vi "Overlay Coordinate System.vi"(6 "Color":u32(colorbox)=16711680, 7 "Group":string, 8 "error in":errorcluster, 9 "Axis Length":i32=150, 10 "Calibration Axis Info":T2={"Origin Pixel"={"X"=0.0, "Y"=0.0}, "Angle Relative to Horizontal (deg)"=20.0, "Axis Reference"=0} {"Axis Reference" items=["Direct", "Indirect"]; "Angle Relative to Horizontal (deg)" format="%.2f"}, 11 "Image":T1) -> (0 "error out":errorcluster, 3 "Image Out":T1)   [LabVIEW 2016]
doc: "Overlay a coordinate system on the image."
uses:
  <vilib>/vision/Image Controls.llb/IMAQ Image.ctl
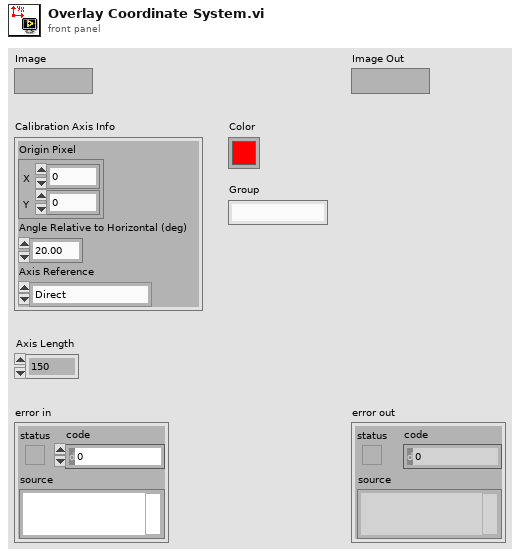
[diagram p1: front panel]
types:
  T1 = typedef "IMAQ Image.ctl" = refnum<image>
  T2 = cluster{"Origin Pixel":cluster{"X":sgl, "Y":sgl}, "Angle Relative to Horizontal (deg)":sgl, "Axis Reference":u32}
  T3 = cluster{"Origin Pixel":cluster{"X":dbl, "Y":dbl}, "Angle Relative to Horizontal (deg)":dbl, "Axis Reference":dbl}
  T4 = cluster{"[0]":dbl, "[1]":dbl, "[2]":dbl, "[3]":dbl}
  T5 = cluster{"[0]":i32, "[1]":i32, "[2]":i32, "[3]":i32}
  T6 = cluster{"Origin Pixel":cluster{"X":dbl, "Y":dbl}, cluster{dbl, dbl}}
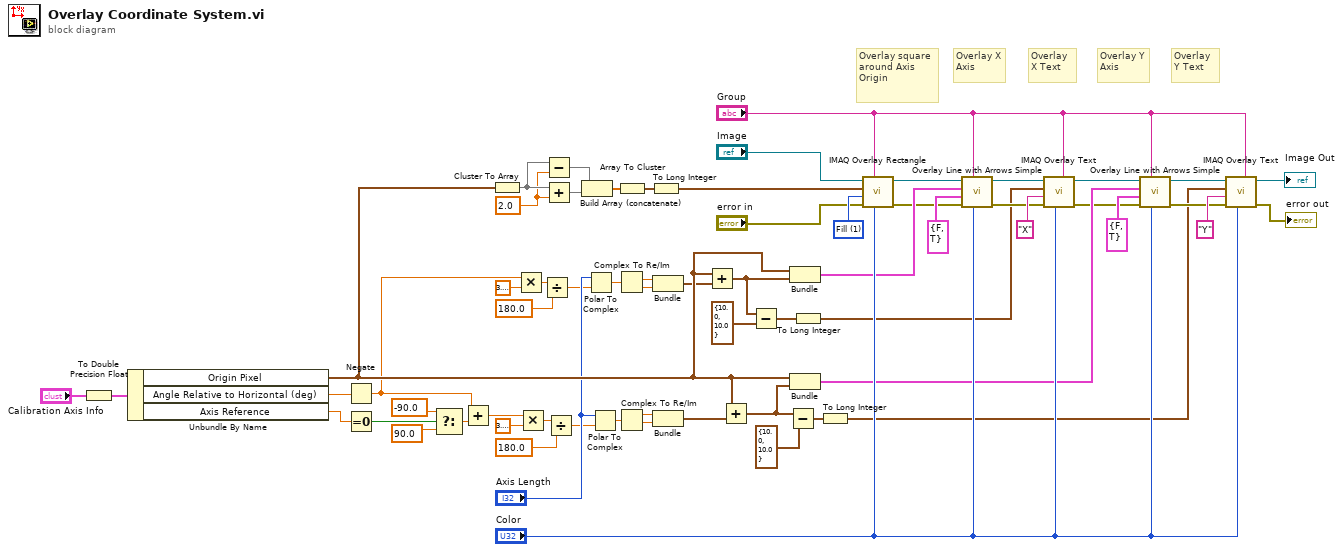
[diagram p0: block diagram]
diagram:
  w49 = u32 1 items=["Frame", "Fill", "Highlight"] ("Drawing Mode (Frame)")
  w54 = 2.0
  # "Overlay Y Text"
  # "Overlay Y Axis"
  # "Overlay X Text"
  # "Overlay X Axis"
  # "Overlay square around Axis Origin"
  n1 = To Double Precision Float(number="Calibration Axis Info") -> (double precision float=w11:T3)
  n2 = Unbundle By Name(w11) -> ("Origin Pixel"=w59:cluster{"X":dbl, "Y":dbl}, "Angle Relative to Horizontal (deg)"=w62:dbl, "Axis Reference"=w57:dbl)
  n3 = Negate(x=w62) -> (-x=w12:dbl)
  n4 = Equal To 0?(x=w57) -> (x = 0?=w23:bool)
  n5 = Select(t=-90.0, s=w23, f=90.0 ("t")) -> (s? t:f=w20:dbl)
  n6 = Add(x=w12, y=w20) -> (x+y=w19:dbl)
  n7 = Cluster To Array(cluster=w59) -> (array=w55:dbl[])
  n8 = Multiply(x=w12, y=3.141592653589793) -> (x*y=w47:dbl)
  n9 = Multiply(x=w19, y=3.141592653589793) -> (x*y=w32:dbl)
  n10 = Divide(x=w47, y=180.0) -> (x/y=w45:dbl)
  n11 = Subtract(x=w55, y=w54) -> (x-y=w53:dbl[])
  n12 = Add(x=w55, y=w54) -> (x+y=w52:dbl[])
  n13 = Divide(x=w32, y=180.0) -> (x/y=w30:dbl)
  n14 = Build Array (concatenate)(w53, w52) -> (w51:dbl[])
  n15 = Polar To Complex(1:w45, 2:"Axis Length") -> (0:w44:cdb)
  n16 = Polar To Complex(1:w30, 2:"Axis Length") -> (0:w29:cdb)
  n17 = Array To Cluster(array=w51) -> (cluster=w50:T4)
  n18 = Complex To Re/Im(x + iy=w44) -> (x=w43:dbl, y=w42:dbl)
  n19 = Complex To Re/Im(x + iy=w29) -> (x=w28:dbl, y=w27:dbl)
  n20 = To Long Integer(number=w50) -> (32bit integer=w10:T5)
  n21 = Bundle(w43, w42) -> (w41:cluster{dbl, dbl})  [unwired: 1 out]
  n22 = Bundle(w28, w27) -> (w26:cluster{dbl, dbl})  [unwired: 1 out]
  n23 = Add(x=w59, y=w41) -> (x+y=w37:cluster{dbl, dbl})
  n24 = Add(x=w59, y=w26) -> (x+y=w16:cluster{dbl, dbl})
  n25 = Subtract(x=w37, y=cluster{dbl, dbl} {10.0, 10.0}) -> (x-y=w36:cluster{dbl, dbl})
  n26 = Subtract(x=w16, y=cluster{dbl, dbl} {10.0, 10.0}) -> (x-y=w13:cluster{dbl, dbl})
  n27 = Bundle("Origin Pixel"=w59, w37) -> (w40:T6)  [unwired: 1 out]
  n28 = Bundle("Origin Pixel"=w59, w16) -> (w25:T6)  [unwired: 1 out]
  n29 = To Long Integer(number=w36) -> (32bit integer=w2:cluster{i32, i32})
  n30 = To Long Integer(number=w13) -> (32bit integer=w1:cluster{i32, i32})
  n31 = call "IMAQ Overlay Rectangle"("Color"="Color", "Group"="Group", "error in (no error)"="error in", "Drawing Mode (Frame)"=w49, "Rectangle"=w10, "Image"="Image") -> ("error out"=w6:errorcluster, "Image Out"=w61:T1)  [unwired: 4 out]
  n32 = call "Overlay Line with Arrows Simple.vi"("Color"="Color", "Group"="Group", "error in"=w6, "Arrows"=cluster{"Start point":bool, "End point":bool} {"Start point"=FALSE, "End point"=TRUE}, "Line Coordinates"=w40, "Image In"=w61) -> ("error out"=w7:errorcluster, "Image Out"=w38:T1)  [unwired: 4 in]
  n33 = call "IMAQ Overlay Text"("Group"="Group", "Text Color (black)"="Color", "error in (no error)"=w7, "String"="X", "Origin"=w2, "Image"=w38) -> ("error out"=w9:errorcluster, "Image Out"=w56:T1)  [unwired: 2 in, 2 out]
  n34 = call "Overlay Line with Arrows Simple.vi"("Color"="Color", "Group"="Group", "error in"=w9, "Arrows"=cluster{"Start point":bool, "End point":bool} {"Start point"=FALSE, "End point"=TRUE}, "Line Coordinates"=w25, "Image In"=w56) -> ("error out"=w8:errorcluster, "Image Out"=w17:T1)  [unwired: 4 in]
  n35 = call "IMAQ Overlay Text"("Group"="Group", "Text Color (black)"="Color", "error in (no error)"=w8, "String"="Y", "Origin"=w1, "Image"=w17) -> ("error out"=→"error out":errorcluster, "Image Out"=→"Image Out":T1)  [unwired: 2 in, 2 out]
